vi "XIPIN_LTE_UL_Channel_Decoder_4_0.vi"   [LabVIEW 2017]
doc: "The Xilinx IP LTE UL Channel Decoder implements an AXI4 compliant, high-performance, optimized block for the 3GPP TS 36.212 v9.3.0 uplink shared channel.\n------------------------------------\n<b>Need License</b> : Yes\n<b>Interface</b> : AXI4 AXI4-Stream"
uses:
  <vilib>/rvi/XilinxIP/XIPIN_XNode/niFpgaXIPIN.xnode
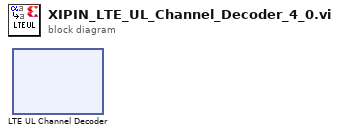
[diagram p0: block diagram]
diagram:
  n1 = xnode ("LTE UL Channel Decoder")() -> ()
